vi "Edge Inspect.vi"(7 "Process":T4(ring)=enum."Get Best Edge", 8 "error in (no error)":errorcluster, 9 "Edge Options":T1={"Edge Polarity"=0, "Kernel Size"=3, "Width"=3, "Minimum Edge Strength"=10.0, "Interpolation Type"=enum."Bilinear Fixed", "Data Processing Method"=enum."Average"} {"Edge Polarity" items=["All Edges", "Rising Edges", "Falling Edges"]; "Minimum Edge Strength" format="%.2f"; "Width" step=2; "Kernel Size" step=2}, 10 "ROI Descriptor":T6 {"Contours"."Type" items=["No Selection", "Point", "Line", "Rectangle", "Oval", "Polygon", "Freehand Region", "Annulus", "Unused2", "Unused3", "Broken Line", "Freehand Line", "Rotated Rectangle"]}, 11 "Main_RGB":T3) -> (0 "error out":errorcluster, 1 "Edge Information":T5[](array[typedef]) {"Distance (Real-World)" format="%.2f"; "Location (Real-World)"."Y" format="%.2g"; "Location (Real-World)"."X" format="%.2f"; "Noise" format="%.2f"; "Location (Pixel)"."Y" format="%.2g"; "Location (Pixel)"."X" format="%.2f"; "Strength" format="%.2f"; "Distance (Pixel)" format="%.2f"}, 2 "Number of Edges":i32, 3 "Image":T3(plugin-control))   [LabVIEW 2020]
uses:
  <vilib>/vision/Image Controls.llb/IMAQ Image.ctl
  <vilib>/vision/Measure.llb/Edge New.ctl
  <vilib>/vision/Measure.llb/Edge Options.ctl
  <vilib>/vision/Measure.llb/Edge Polarity.ctl
  <vilib>/vision/NI_Vision_Development_Module.lvlib
panel:
  out "Image 2":T3(plugin-control)
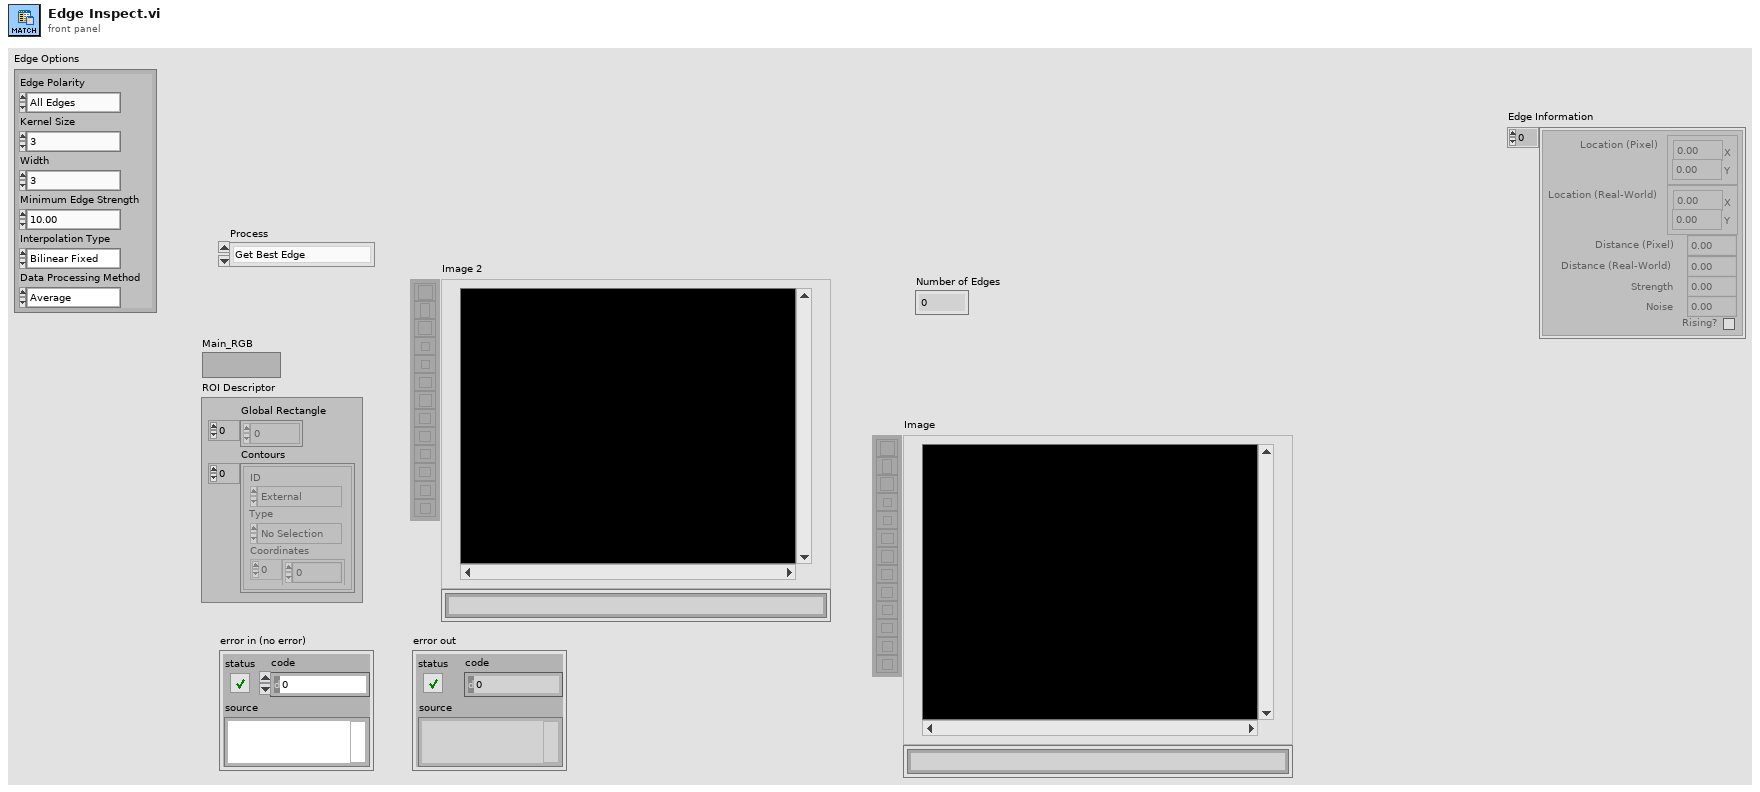
[diagram p1: front panel]
types:
  T1 = typedef "Edge Options.ctl" = cluster{"Edge Polarity":T2, "Kernel Size":u32, "Width":u32, "Minimum Edge Strength":sgl, "Interpolation Type":enum32{"Zero Order", "Bilinear", "Quadratic", "Cubic", "Bilinear Fixed"}, "Data Processing Method":enum32{"Average", "Median"}}
  T2 = typedef "Edge Polarity.ctl" = u32
  T3 = typedef "IMAQ Image.ctl" = refnum<image>
  T4 = enum16{"Get First Edge", "Get First + Last Edge", "Get All Edges", "Get Best Edge"}
  T5 = typedef "Edge New.ctl" = cluster{"Location (Pixel)":cluster{"X":sgl, "Y":sgl}, "Location (Real-World)":cluster{"X":sgl, "Y":sgl}, "Distance (Pixel)":dbl, "Distance (Real-World)":dbl, "Strength":dbl, "Noise":dbl, "Rising?":bool}
  T6 = typedef "ROI Descriptor" = cluster{"Global Rectangle":i32[], "Contours":cluster{"ID":enum32{"External", "Internal"}, "Type":u32, "Coordinates":i32[]}[]}
  T7 = typedef "IMAQ Line" = cluster{"Start X":i32, "Start Y":i32, "End X":i32, "End Y":i32}
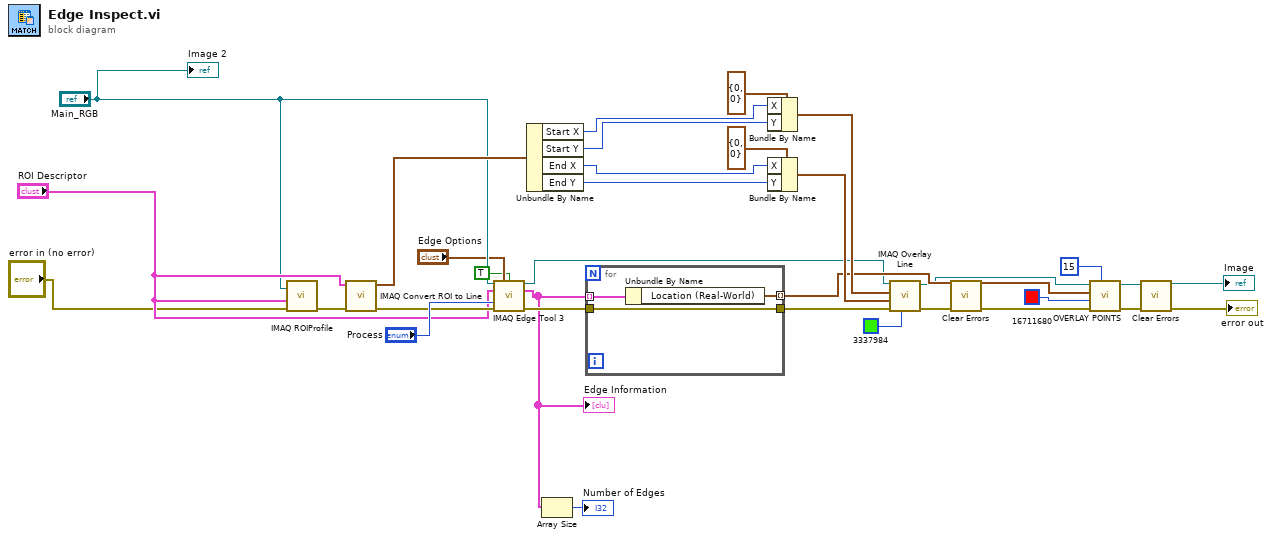
[diagram p0: block diagram]
diagram:
  n1 = call "IMAQ ROIProfile"("error in (no error)"="error in (no error)", "ROI Descriptor"="ROI Descriptor", "Image"="Main_RGB") -> ("error out"=w21:errorcluster)  [unwired: 1 in, 4 out]
  n2 = call "IMAQ Convert ROI to Line"("error in (no error)"=w21, "ROI Descriptor"="ROI Descriptor") -> ("error out"=w20:errorcluster, "Line"=w19:T7)  [unwired: 7 in]
  n3 = call "IMAQ Edge Tool 3"("Image"="Main_RGB", "Edge Options"="Edge Options", "Optimized Mode"=TRUE, "ROI Descriptor"="ROI Descriptor", "Process"="Process", "error in (no error)"=w20) -> ("Image (duplicate)"=w10:T3, "Edge Information"=w7:T5[], "error out"=w32:errorcluster)  [unwired: 5 in, 2 out]
  "Edge Information" <- w7
  n4 = Unbundle By Name(w19) -> ("Start X"=w29:i32, "Start Y"=w28:i32, "End X"=w24:i32, "End Y"=w23:i32)
  n5 = Array Size(array=w7) -> (size(s)=→"Number of Edges":i32)
  n6 = for {
    tunnel: w7 -> [w35] mode=indexing
    tunnel: [w34] -> w16 mode=indexing
    tunnel: w32 -> [w33]
    tunnel: [w33] -> w17
    n7 = Unbundle By Name(w35) -> ("Location (Real-World)"=w34:cluster{"X":sgl, "Y":sgl})
  }
  n8 = Bundle By Name(cluster=cluster{"X":i32, "Y":i32} {"X"=0, "Y"=0} ("End Point"), "X"=w29, "Y"=w28) -> (w27:cluster{"X":i32, "Y":i32})
  n9 = Bundle By Name(cluster=cluster{"X":i32, "Y":i32} {"X"=0, "Y"=0} ("End Point"), "X"=w24, "Y"=w23) -> (w25:cluster{"X":i32, "Y":i32})
  n10 = call "IMAQ Overlay Line"("Color"=u32 3337984, "error in (no error)"=w17, "End Point"=w25, "Start Point"=w27, "Image"=w10) -> ("error out"=w18:errorcluster, "Image Out"=w15:T3)  [unwired: 5 in]
  n11 = call <vilib>:"Clear Errors.vi"("error in (no error)"=w18) -> ("error out"=w14:errorcluster)  [unwired: 5 in, 1 out]
  n12 = call "OVERLAY POINTS.vi"("Point Diameter (5)"=u32 15, "error in"=w14, "Color"=u32 16711680, "Points"=w16, "Image In"=w15) -> ("error out"=w5:errorcluster, "Image Out"=→"Image":T3)  [unwired: 5 in]
  n13 = call <vilib>:"Clear Errors.vi"("error in (no error)"=w5) -> ("error out"=→"error out":errorcluster)  [unwired: 5 in, 1 out]
  "Image 2" <- "Main_RGB"
